vi "Position Z Key.vi"(8 "error in (no error)":errorcluster, 10 "A Key":refnum<vi>, 11 "Z Key":refnum<vi>) -> (0 "error out":errorcluster)   [LabVIEW 2014]
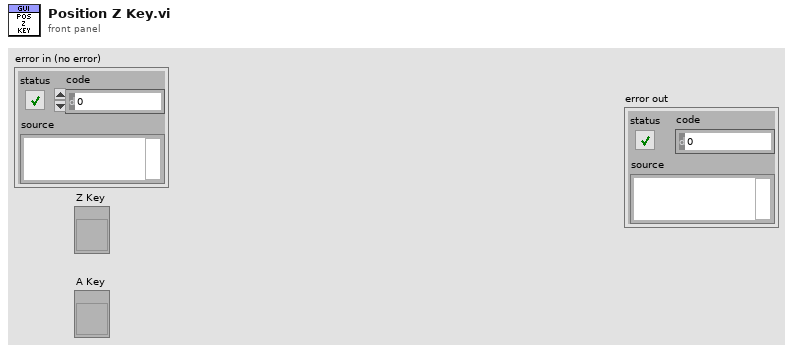
[diagram p1: front panel]
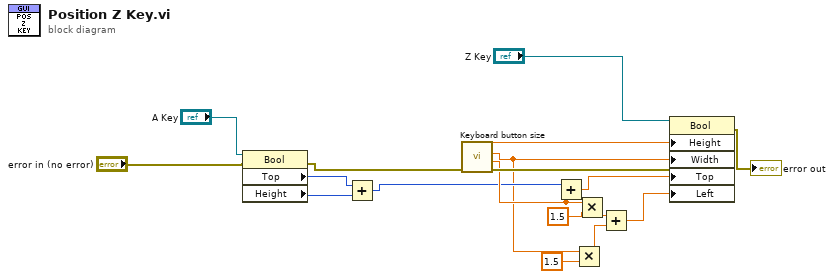
[diagram p0: block diagram]
diagram:
  n1 = property class="Bool"(reference="A Key", error in="error in (no error)") -> (error out=w12:errorcluster, "Top"=w10:i32, "Height"=w9:u32)  [unwired: 1 out]
  n2 = Add(x=w10, y=w9) -> (x+y=w7:u32)
  n3 = call "Keyboard button size.vi"("error in (no error)"=w12) -> ("error out"=w17:errorcluster, "Key Spacing"=w8:dbl, "Key Width"=w3:dbl, "Key Height"=w15:dbl)  [unwired: 7 in]
  n4 = Add(x=w7, y=w8) -> (x+y=w6:dbl)
  n5 = Multiply(x=w3, y=1.5) -> (x*y=w1:dbl)
  n6 = Multiply(x=w8, y=1.5) -> (x*y=w5:dbl)
  n7 = Add(x=w5, y=w1) -> (x+y=w4:dbl)
  n8 = property class="Bool"(reference="Z Key", error in=w17, "Height"=w15, "Width"=w3, "Top"=w6, "Left"=w4) -> (error out=→"error out":errorcluster)  [unwired: 1 out]
